vi "OutputSwerveAzimuth2.vi"() -> ()   [LabVIEW 2019]
doc: "This VI runs feedback and feedforward control loops, manages safety interlocks, and sends commands to the swerve azimuth motors."
uses:
  <vilib>/Rock Robotics/WPI/ThirdParty/Phoenix-LabVIEW/Motor Controller/Controls/CTRE_Phoenix_MotorControl_ControlMode.ctl
  refnums.vi
  GRNF_CTREMotor.vi
  outputs.vi
  sensors.vi
  TAI_Motor.vi
  dsdata.vi
panel:
  in  "Overriden Azimuth Goal (deg) [-180,180]":dbl
  in  "Manually Override Azimuth Goal":bool
  in  "Best Angle Hysteresis (deg)":dbl=20.0 format="%#_13g"
  in  "PID Parameters Module 3":T1={"Kp"=0.002, "Ki"=0.003, "Kd"=0.00015, "N-Diff"=10, "N-Int"=10, "Int Error Window"=20.0, "Max Ouput"=1.0, "Min Output"=-1.0} {"Int Error Window" min=0.0; "N-Int" min=2; "N-Diff" min=2; "Kd" min=0.0; "Ki" min=0.0; "Kp" min=0.0}
  in  "PID Parameters Module 2":T1={"Kp"=0.002, "Ki"=0.003, "Kd"=0.00015, "N-Diff"=10, "N-Int"=10, "Int Error Window"=20.0, "Max Ouput"=1.0, "Min Output"=-1.0} {"Int Error Window" min=0.0; "N-Int" min=2; "N-Diff" min=2; "Kd" min=0.0; "Ki" min=0.0; "Kp" min=0.0}
  in  "PID Parameters Module 1":T1={"Kp"=0.002, "Ki"=0.003, "Kd"=0.00015, "N-Diff"=10, "N-Int"=10, "Int Error Window"=20.0, "Max Ouput"=1.0, "Min Output"=-1.0} {"Int Error Window" min=0.0; "N-Int" min=2; "N-Diff" min=2; "Kd" min=0.0; "Ki" min=0.0; "Kp" min=0.0}
  in  "Plotting":T2(ring)
  out "Controller Summary":T3(graph)
  in  "PID Parameters Module 0":T1={"Kp"=0.002, "Ki"=0.003, "Kd"=0.00015, "N-Diff"=10, "N-Int"=10, "Int Error Window"=20.0, "Max Ouput"=1.0, "Min Output"=-1.0} {"Int Error Window" min=0.0; "N-Int" min=2; "N-Diff" min=2; "Kd" min=0.0; "Ki" min=0.0; "Kp" min=0.0}
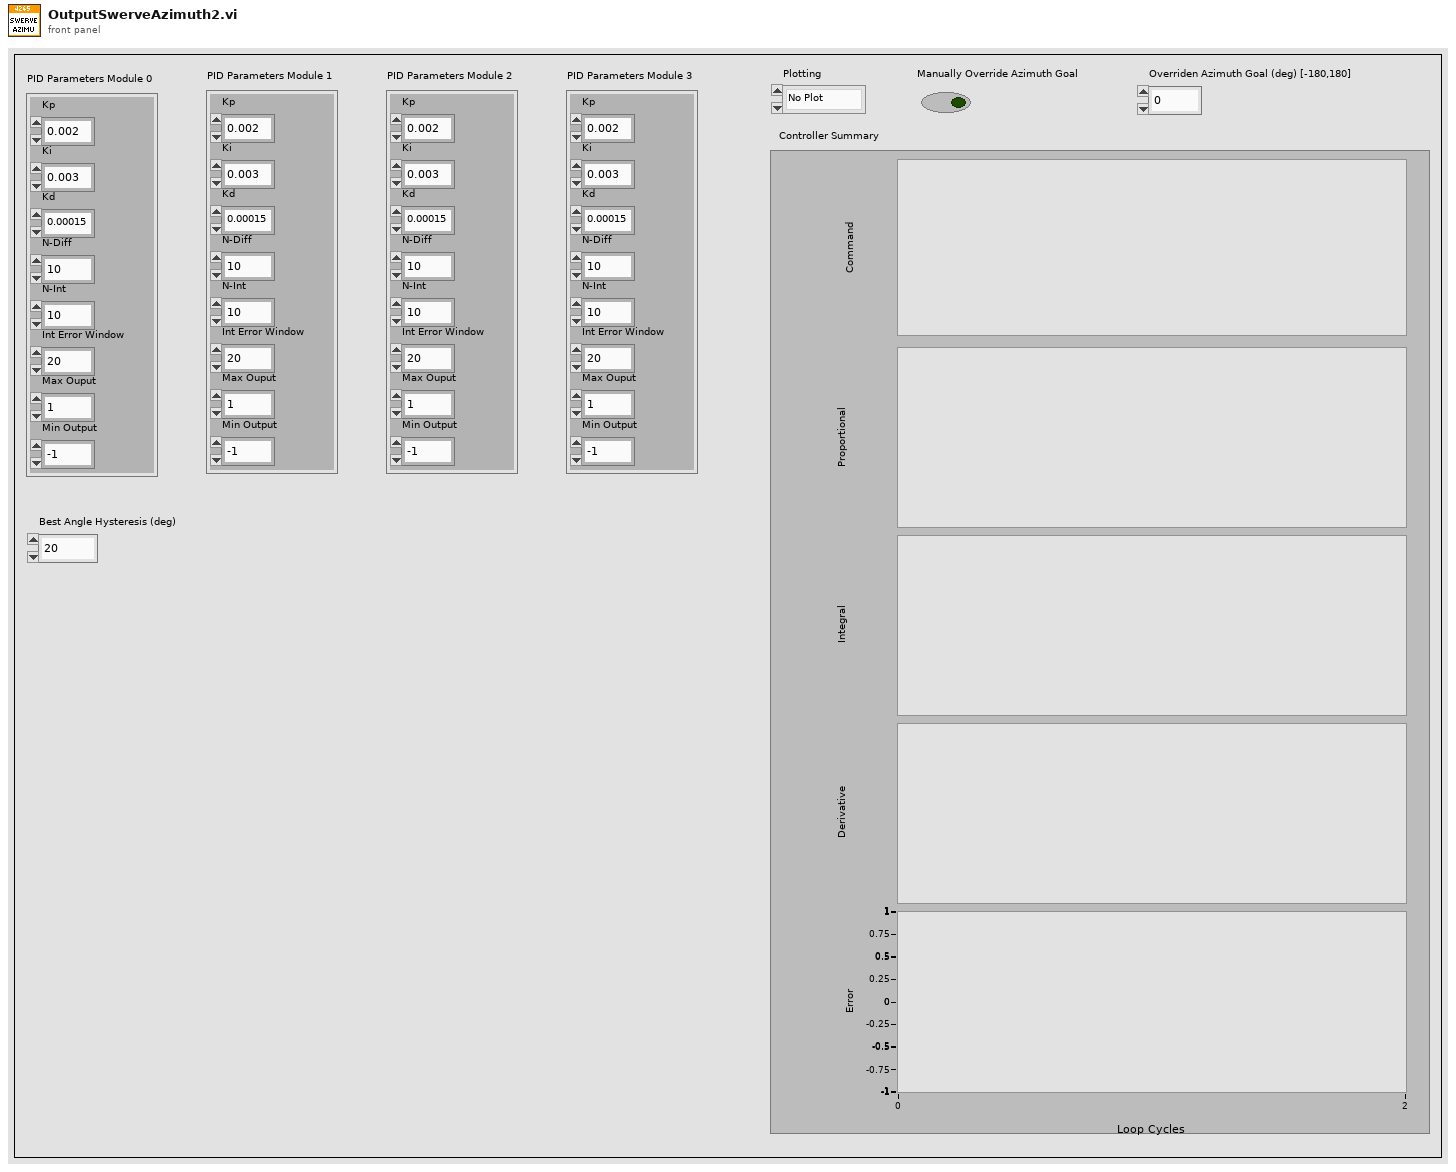
[diagram p1: front panel]
types:
  T1 = cluster{"Kp":dbl, "Ki":dbl, "Kd":dbl, "N-Diff":i32, "N-Int":i32, "Int Error Window":dbl, "Max Ouput":dbl, "Min Output":dbl}
  T2 = enum16{"No Plot", "Module 0", "Module 1", "Module 2", "Module 3"}
  T3 = cluster{"Command":dbl, "Proportional":dbl, "Integral":dbl, "Derivative":dbl, "Goal":dbl}
  T4 = typedef "CTRE_Phoenix_MotorControl_ControlMode.ctl" = u16
  T5 = typedef "WPI_MotorControlDeviceRef.ctl" = cluster{"DeviceStatus":errorcluster, "Type":T6, "PWM":cluster{"PWM Channel":T7, "DeadBand":T8}, "CAN":cluster{"Device Number":u8, "SetOutput VI Ref":variant, "GetOutput VI Ref":variant, "Enable VI Ref":variant, "Disable VI Ref":variant, "Data":variant}, "Invert":bool, "DIO PWM":cluster{"PWM \"Enable\" Channel":T7, "DIOChannel":T9, "PWM Rate":dbl}}
  T6 = typedef "WPI_MotorControlType.ctl" = enum16{"PWM", "CAN", "DIO PWM"}
  T7 = typedef "FPGA_DIOPWMChannel.ctl" = enum8{"PWM 0", "PWM 1", "PWM 2", "PWM 3", "PWM 4", "PWM 5", "PWM 6", "PWM 7", "PWM 8", "PWM 9", "PWM MXP 0", "PWM MXP 1", "PWM MXP 2", "PWM MXP 3", "PWM MXP 4", "PWM MXP 5", "PWM MXP 6", "PWM MXP 7", "PWM MXP 8", "PWM MXP 9", "Invalid"}
  T8 = typedef "WPI_PWMDeadband.ctl" = cluster{"Name":string, "maxPositivePwm":i32, "minPositivePwm":i32, "centerPwm":i32, "maxNegativePwm":i32, "minNegativePwm":i32, "angularRange":u16}
  T9 = typedef "FPGA_DIOChannel.ctl" = enum8{"DIO 0", "DIO 1", "DIO 2", "DIO 3", "DIO 4", "DIO 5", "DIO 6", "DIO 7", "DIO 8", "DIO 9", "DIO MXP 0", "DIO MXP 1", "DIO MXP 2", "DIO MXP 3", "DIO MXP 4", "DIO MXP 5", "DIO MXP 6", "DIO MXP 7", "DIO MXP 8", "DIO MXP 9", "DIO MXP 10", "DIO MXP 11", "DIO MXP 12", "DIO MXP 13", "DIO MXP 14", "DIO MXP 15", "SPI Port CS1", "SPI Port CS2", "SPI Port CS3", "SPI Port MISO", "SPI Port MOSI", "Invalid"}
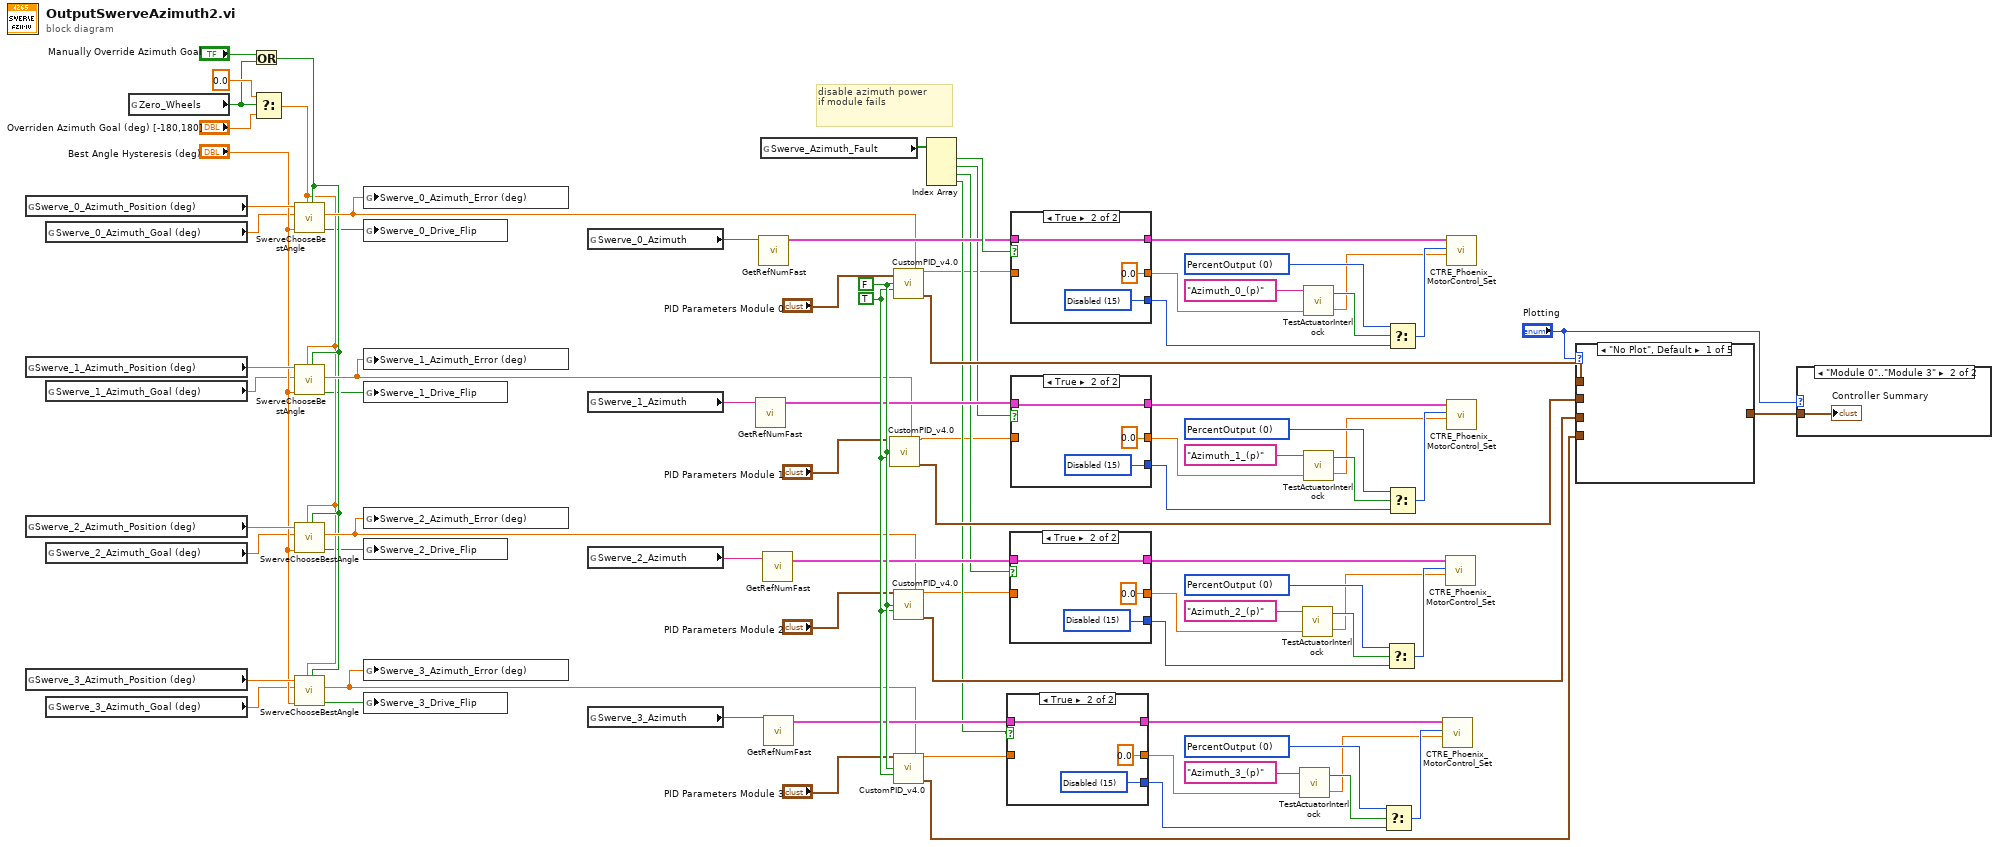
[diagram p0: block diagram]
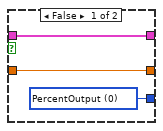
[diagram p2: hidden frame]
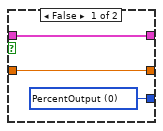
[diagram p3: hidden frame]
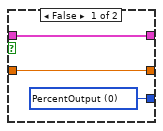
[diagram p4: hidden frame]
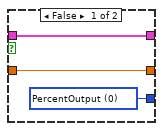
[diagram p10: hidden frame]
diagram:
  w37 = T4 0 items=["PercentOutput"=0, "Position"=1, "Velocity"=2, "Current"=3, "Follower"=5, "MotionProfile"=6, "MotionMagic"=7, "MotionProfileArc"=10, "Disabled"=15] ("Control Mode")
  w48 = T4 0 items=["PercentOutput"=0, "Position"=1, "Velocity"=2, "Current"=3, "Follower"=5, "MotionProfile"=6, "MotionMagic"=7, "MotionProfileArc"=10, "Disabled"=15] ("Control Mode")
  w58 = T4 0 items=["PercentOutput"=0, "Position"=1, "Velocity"=2, "Current"=3, "Follower"=5, "MotionProfile"=6, "MotionMagic"=7, "MotionProfileArc"=10, "Disabled"=15] ("Control Mode")
  w66 = T4 0 items=["PercentOutput"=0, "Position"=1, "Velocity"=2, "Current"=3, "Follower"=5, "MotionProfile"=6, "MotionMagic"=7, "MotionProfileArc"=10, "Disabled"=15] ("Control Mode")
  w76 = FALSE ("Reset on Goal Change ?")
  w75 = TRUE ("Use Custom Error Calculation ?")
  # "disable azimuth power\nif module fails"
  n1 = global read "sensors.vi" "Swerve_0_Azimuth_Position (deg)"() -> (w15:dbl)
  n2 = global read "sensors.vi" "Swerve_1_Azimuth_Position (deg)"() -> (w14:dbl)
  n3 = global read "sensors.vi" "Swerve_2_Azimuth_Position (deg)"() -> (w13:dbl)
  n4 = global read "sensors.vi" "Swerve_3_Azimuth_Position (deg)"() -> (w12:dbl)
  n5 = global read "outputs.vi" "Swerve_0_Azimuth_Goal (deg)"() -> (w8:dbl)
  n6 = global read "outputs.vi" "Swerve_1_Azimuth_Goal (deg)"() -> (w7:dbl)
  n7 = global read "outputs.vi" "Swerve_2_Azimuth_Goal (deg)"() -> (w6:dbl)
  n8 = global read "outputs.vi" "Swerve_3_Azimuth_Goal (deg)"() -> (w5:dbl)
  n9 = global read "dsdata.vi" "Zero_Wheels"() -> (w20:bool)
  n10 = Or(x="Manually Override Azimuth Goal", y=w20) -> (x .or. y?=w11:bool)
  n11 = Select(t=0.0 ("f"), s=w20, f="Overriden Azimuth Goal (deg) [-180,180]") -> (s? t:f=w10:dbl)
  n12 = call "SwerveChooseBestAngle.vi"("Goal Override"=w11, "Goal Override Angle (deg) [-180,+180]"=w10, "Hysteresis (deg)"="Best Angle Hysteresis (deg)", "Goal Angle (deg) [-180,+180]"=w8, "Current Angle (deg) [-180,+180]"=w15) -> ("Flip Drive Motor Direction"=w4:bool, "Angular Distance (deg)"=w19:dbl)  [unwired: 5 in]
  n13 = call "SwerveChooseBestAngle.vi"("Goal Override"=w11, "Goal Override Angle (deg) [-180,+180]"=w10, "Hysteresis (deg)"="Best Angle Hysteresis (deg)", "Goal Angle (deg) [-180,+180]"=w7, "Current Angle (deg) [-180,+180]"=w14) -> ("Flip Drive Motor Direction"=w3:bool, "Angular Distance (deg)"=w18:dbl)  [unwired: 5 in]
  n14 = call "SwerveChooseBestAngle.vi"("Goal Override"=w11, "Goal Override Angle (deg) [-180,+180]"=w10, "Hysteresis (deg)"="Best Angle Hysteresis (deg)", "Goal Angle (deg) [-180,+180]"=w6, "Current Angle (deg) [-180,+180]"=w13) -> ("Flip Drive Motor Direction"=w2:bool, "Angular Distance (deg)"=w17:dbl)  [unwired: 5 in]
  n15 = call "SwerveChooseBestAngle.vi"("Goal Override"=w11, "Goal Override Angle (deg) [-180,+180]"=w10, "Hysteresis (deg)"="Best Angle Hysteresis (deg)", "Goal Angle (deg) [-180,+180]"=w5, "Current Angle (deg) [-180,+180]"=w12) -> ("Flip Drive Motor Direction"=w1:bool, "Angular Distance (deg)"=w16:dbl)  [unwired: 5 in]
  n16 = global write "outputs.vi" "Swerve_0_Azimuth_Error (deg)"(w19) -> ()
  n17 = global write "outputs.vi" "Swerve_0_Drive_Flip"(w4) -> ()
  n18 = global write "outputs.vi" "Swerve_1_Azimuth_Error (deg)"(w18) -> ()
  n19 = global write "outputs.vi" "Swerve_1_Drive_Flip"(w3) -> ()
  n20 = global write "outputs.vi" "Swerve_2_Azimuth_Error (deg)"(w17) -> ()
  n21 = global write "outputs.vi" "Swerve_2_Drive_Flip"(w2) -> ()
  n22 = global write "outputs.vi" "Swerve_3_Azimuth_Error (deg)"(w16) -> ()
  n23 = global write "outputs.vi" "Swerve_3_Drive_Flip"(w1) -> ()
  n24 = global read "refnums.vi" "Swerve_0_Azimuth"() -> (w81:string)
  n25 = global read "refnums.vi" "Swerve_1_Azimuth"() -> (w80:string)
  n26 = global read "refnums.vi" "Swerve_2_Azimuth"() -> (w79:string)
  n27 = global read "refnums.vi" "Swerve_3_Azimuth"() -> (w78:string)
  n28 = call-poly "GetRefNumFast.vi"("RefNum Name"=w80) -> ("Device Reference"=w53:T5)  [unwired: 5 in, 1 out]
  n29 = call-poly "GetRefNumFast.vi"("RefNum Name"=w81) -> ("Device Reference"=w82:T5)  [unwired: 5 in, 1 out]
  n30 = global read "sensors.vi" "Swerve_Azimuth_Fault"() -> (w83:bool[])
  n31 = call-poly "GetRefNumFast.vi"("RefNum Name"=w79) -> ("Device Reference"=w43:T5)  [unwired: 5 in, 1 out]
  n32 = call-poly "GetRefNumFast.vi"("RefNum Name"=w78) -> ("Device Reference"=w32:T5)  [unwired: 5 in, 1 out]
  n33 = call "CustomPID_v4.0.vi"("PID Tuning Parameters"="PID Parameters Module 1", "Custom Error Calculation"=w18, "Reset on Goal Change ?"=w76, "Use Custom Error Calculation ?"=w75) -> ("Command"=w28:dbl, "Controller Summary"=w71:T3)  [unwired: 8 in, 2 out]
  n34 = call "CustomPID_v4.0.vi"("PID Tuning Parameters"="PID Parameters Module 0", "Custom Error Calculation"=w19, "Reset on Goal Change ?"=w76, "Use Custom Error Calculation ?"=w75) -> ("Command"=w27:dbl, "Controller Summary"=w72:T3)  [unwired: 8 in, 2 out]
  n35 = call "CustomPID_v4.0.vi"("PID Tuning Parameters"="PID Parameters Module 2", "Custom Error Calculation"=w17, "Reset on Goal Change ?"=w76, "Use Custom Error Calculation ?"=w75) -> ("Command"=w29:dbl, "Controller Summary"=w41:T3)  [unwired: 8 in, 2 out]
  n36 = call "CustomPID_v4.0.vi"("PID Tuning Parameters"="PID Parameters Module 3", "Custom Error Calculation"=w16, "Reset on Goal Change ?"=w76, "Use Custom Error Calculation ?"=w75) -> ("Command"=w30:dbl, "Controller Summary"=w70:T3)  [unwired: 8 in, 2 out]
  n37 = Index Array(array=w83) -> (element #1=w84:bool, element #2=w52:bool, element #3=w42:bool, element #4=w31:bool)  [unwired: 4 in]
  n38 = case shown="True" w31 {
    tunnel: [w87 w90] -> w40
    tunnel: w32 -> [w87 w90]
    tunnel: [w86 0.0 ("Command")] -> w36
    tunnel: w30 -> [w86 _]
    tunnel: [w85 w88] -> w35
    frame False {
      w85 = T4 0 items=["PercentOutput"=0, "Position"=1, "Velocity"=2, "Current"=3, "Follower"=5, "MotionProfile"=6, "MotionMagic"=7, "MotionProfileArc"=10, "Disabled"=15] ("Control Mode")
    }
    frame True {
      w88 = T4 15 items=["PercentOutput"=0, "Position"=1, "Velocity"=2, "Current"=3, "Follower"=5, "MotionProfile"=6, "MotionMagic"=7, "MotionProfileArc"=10, "Disabled"=15] ("Control Mode")
    }
  }
  n39 = case shown="True" w42 {
    tunnel: [w93 w96] -> w51
    tunnel: w43 -> [w93 w96]
    tunnel: [w92 0.0 ("Command")] -> w47
    tunnel: w29 -> [w92 _]
    tunnel: [w91 w94] -> w46
    frame False {
      w91 = T4 0 items=["PercentOutput"=0, "Position"=1, "Velocity"=2, "Current"=3, "Follower"=5, "MotionProfile"=6, "MotionMagic"=7, "MotionProfileArc"=10, "Disabled"=15] ("Control Mode")
    }
    frame True {
      w94 = T4 15 items=["PercentOutput"=0, "Position"=1, "Velocity"=2, "Current"=3, "Follower"=5, "MotionProfile"=6, "MotionMagic"=7, "MotionProfileArc"=10, "Disabled"=15] ("Control Mode")
    }
  }
  n40 = case shown="True" w84 {
    tunnel: [w99 w102] -> w74
    tunnel: w82 -> [w99 w102]
    tunnel: [w98 0.0 ("Command")] -> w65
    tunnel: w27 -> [w98 _]
    tunnel: [w97 w100] -> w64
    frame False {
      w97 = T4 0 items=["PercentOutput"=0, "Position"=1, "Velocity"=2, "Current"=3, "Follower"=5, "MotionProfile"=6, "MotionMagic"=7, "MotionProfileArc"=10, "Disabled"=15] ("Control Mode")
    }
    frame True {
      w100 = T4 15 items=["PercentOutput"=0, "Position"=1, "Velocity"=2, "Current"=3, "Follower"=5, "MotionProfile"=6, "MotionMagic"=7, "MotionProfileArc"=10, "Disabled"=15] ("Control Mode")
    }
  }
  n41 = case shown="True" w52 {
    tunnel: [w105 w108] -> w61
    tunnel: w53 -> [w105 w108]
    tunnel: [w104 0.0 ("Command")] -> w57
    tunnel: w28 -> [w104 _]
    tunnel: [w103 w106] -> w56
    frame False {
      w103 = T4 0 items=["PercentOutput"=0, "Position"=1, "Velocity"=2, "Current"=3, "Follower"=5, "MotionProfile"=6, "MotionMagic"=7, "MotionProfileArc"=10, "Disabled"=15] ("Control Mode")
    }
    frame True {
      w106 = T4 15 items=["PercentOutput"=0, "Position"=1, "Velocity"=2, "Current"=3, "Follower"=5, "MotionProfile"=6, "MotionMagic"=7, "MotionProfileArc"=10, "Disabled"=15] ("Control Mode")
    }
  }
  n42 = call-poly "TestActuatorInterlock.vi"("Normal Output"=w36, "Actuator Name"="Azimuth_3_(p)" ("Actuator_Name")) -> ("Interlock Output"=w33:dbl, "Testing This Actuator"=w39:bool)  [unwired: 1 in]
  n43 = call-poly "TestActuatorInterlock.vi"("Normal Output"=w47, "Actuator Name"="Azimuth_2_(p)" ("Actuator_Name")) -> ("Interlock Output"=w44:dbl, "Testing This Actuator"=w50:bool)  [unwired: 1 in]
  n44 = call-poly "TestActuatorInterlock.vi"("Normal Output"=w65, "Actuator Name"="Azimuth_0_(p)" ("Actuator_Name")) -> ("Interlock Output"=w62:dbl, "Testing This Actuator"=w68:bool)  [unwired: 1 in]
  n45 = call-poly "TestActuatorInterlock.vi"("Normal Output"=w57, "Actuator Name"="Azimuth_1_(p)" ("Actuator_Name")) -> ("Interlock Output"=w54:dbl, "Testing This Actuator"=w60:bool)  [unwired: 1 in]
  n46 = Select(t=w37, s=w39, f=w35) -> (s? t:f=w34:T4)
  n47 = Select(t=w48, s=w50, f=w46) -> (s? t:f=w45:T4)
  n48 = Select(t=w66, s=w68, f=w64) -> (s? t:f=w63:T4)
  n49 = Select(t=w58, s=w60, f=w56) -> (s? t:f=w55:T4)
  n50 = call <vilib>:"CTRE_Phoenix_MotorControl_Set.vi"("Output"=w33, "Control Mode"=w34, "PhoenixMotorControlDevRef"=w40) -> ()  [unwired: 7 in, 2 out]
  n51 = call <vilib>:"CTRE_Phoenix_MotorControl_Set.vi"("Output"=w44, "Control Mode"=w45, "PhoenixMotorControlDevRef"=w51) -> ()  [unwired: 7 in, 2 out]
  n52 = call <vilib>:"CTRE_Phoenix_MotorControl_Set.vi"("Output"=w62, "Control Mode"=w63, "PhoenixMotorControlDevRef"=w74) -> ()  [unwired: 7 in, 2 out]
  n53 = call <vilib>:"CTRE_Phoenix_MotorControl_Set.vi"("Output"=w54, "Control Mode"=w55, "PhoenixMotorControlDevRef"=w61) -> ()  [unwired: 7 in, 2 out]
  n54 = case shown="\"No Plot\", Default" "Plotting" {
    tunnel: [_ w109 w110 w111 w112] -> w73
    tunnel: w72 -> [_ w109 _ _ _]
    tunnel: w71 -> [_ _ w110 _ _]
    tunnel: w41 -> [_ _ _ w111 _]
    tunnel: w70 -> [_ _ _ _ w112]
    frame "No Plot", Default {
    }
    frame "Module 0" {
    }
    frame "Module 1" {
    }
    frame "Module 2" {
    }
    frame "Module 3" {
    }
  }
  n55 = case shown="\"Module 0\"..\"Module 3\"" "Plotting" {
    tunnel: w73 -> [_ w113]
    frame "No Plot", Default {
    }
    frame "Module 0".."Module 3" {
      "Controller Summary" <- w113
    }
  }
